vi "Set Digital.vi"(0 "connection ID":refnum<k16>, 1 "address":u32, 2 "port":u16, 5 "Digital Number":u16, 7 "Digital State":T1 items=["LOW", "HIGH"], 9 "timeout ms (1000)":i32=1000, 11 "error in (no error)":errorcluster, 12 "mask":u16) -> (4 "connection ID out":refnum<k16>, 6 "received data":string, 15 "error out":errorcluster)   [LabVIEW 2016, in "instr.lvlib"]
doc: "Sets given digital io to given state. This affects the digital IO mode as necessary."
uses:
  instr.lvlib
  IO State.ctl
panel:
  out "Send String":string
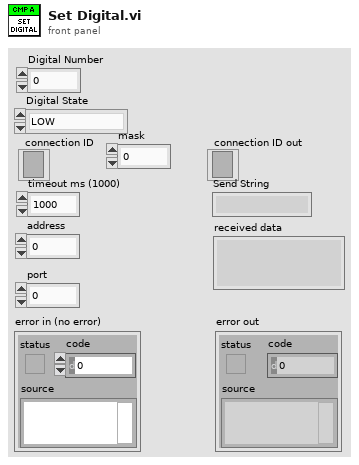
[diagram p1: front panel]
types:
  T1 = typedef "instr.lvlib/IO State.ctl" = u16
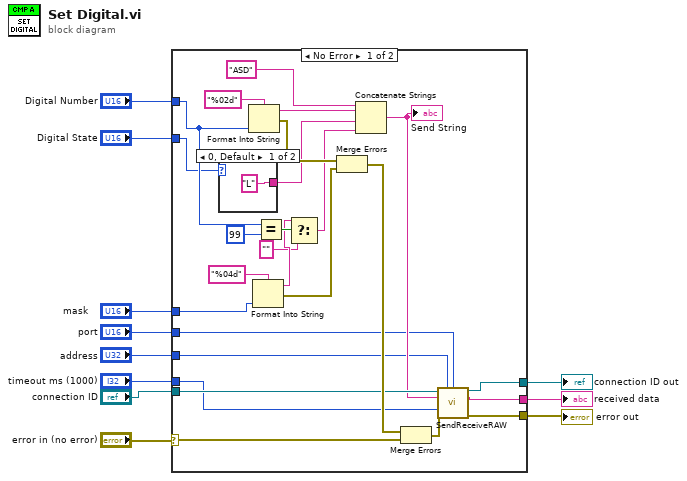
[diagram p0: block diagram]
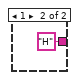
[diagram p2: hidden frame]
diagram:
  n1 = case shown="No Error" "error in (no error)" {
    selector: "error in (no error)" -> [w34 w41]
    tunnel: [w31 w41] -> w11
    tunnel: [w30 _] -> w9
    tunnel: "timeout ms (1000)" -> [w26 _]
    tunnel: "connection ID" -> [w28 w40]
    tunnel: [w29 w40] -> w6
    tunnel: "Digital Number" -> [w17 _]
    tunnel: "Digital State" -> [w14 _]
    tunnel: "address" -> [w24 _]
    tunnel: "port" -> [w23 _]
    tunnel: "mask" -> [w16 _]
    frame No Error {
      n2 = case shown="0, Default" w14 {
        tunnel: ["L" "H"] -> w13
        frame 0, Default {
        }
        frame 1 {
        }
      }
      n3 = Format Into String(format string="%02d", w17) -> (resulting string=w32:string, error out=w35:errorcluster)  [unwired: 2 in]
      n4 = Format Into String(format string="%04d", w16) -> (resulting string=w19:string, error out=w12:errorcluster)  [unwired: 2 in]
      n5 = Equal?(x=w17, y=u16 99) -> (x = y?=w20:bool)
      n6 = Select(t=w19, s=w20, f="") -> (s? t:f=w15:string)
      n7 = Merge Errors(w35, w12) -> (w33:errorcluster)
      n8 = Concatenate Strings("ASD" ("data in"), w32, w13, w15) -> (w25:string)
      "Send String" <- w25
      n9 = Merge Errors(w33, w34) -> (w27:errorcluster)
      n10 = call "SendReceiveRAW.vi"("connection ID"=w28, "address"=w24, "port"=w23, "RAW data in"=w25, "timeout ms (1000)"=w26, "error in (no error)"=w27) -> ("connection ID out"=w29:refnum<k16>, "received data"=w30:string, "error out"=w31:errorcluster)  [unwired: 7 in]
    }
    frame Error {
    }
  }
  "error out" <- w11
  "received data" <- w9
  "connection ID out" <- w6
